vi "OnDataChange.vi"(0 "DemoMicrosope in":refnum<class "DemoMicrosope.lvclass">, 1 "DataExchange":T1, 3 "error in (no error)":errorcluster) -> (7 "DemoMicrosope out":refnum<class "DemoMicrosope.lvclass">, 10 "error out":errorcluster)   [LabVIEW 2020]
uses:
  Hardware Abstraction Layer/Component/Device/Device/DataExchange.ctl
  Interface/DataListener/DataListener.lvclass
  DemoMicrosope.lvclass
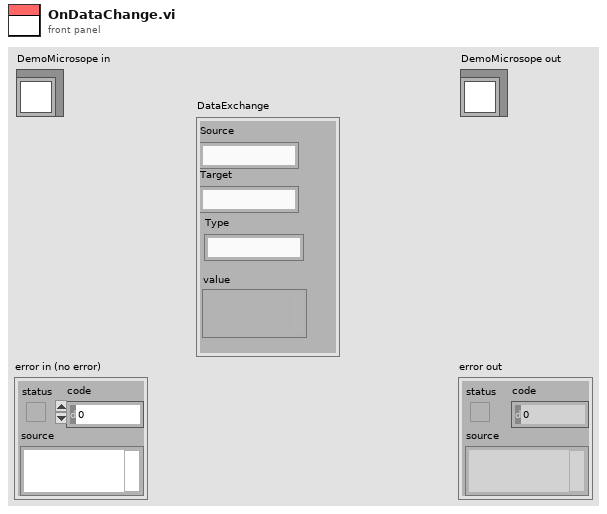
[diagram p1: front panel]
types:
  T1 = typedef "DataListener.lvclass/DataExchange.ctl" = cluster{"Source":string, "Target":string, "Type":string, "value":variant}
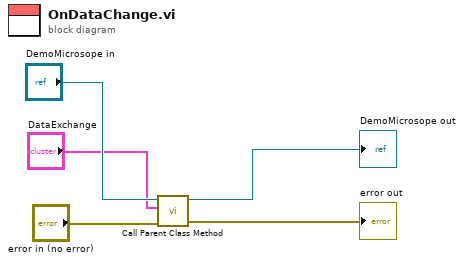
[diagram p0: block diagram]
diagram:
  n1 = call-parent "Call Parent Class Method"("Microscope in"="DemoMicrosope in", "DataExchange"="DataExchange", "error in (no error)"="error in (no error)") -> ("Microscope out"=→"DemoMicrosope out":refnum<class "DemoMicrosope.lvclass">, "error out"=→"error out":errorcluster)  [unwired: 6 in]
